vi "Set Port Interface Name.vi"(8 "error in":errorcluster, 10 "XNET Interface Name":T2, 11 "Port Ref":T1 format="%.0x") -> (0 "error out":errorcluster, 3 "Port Ref out":T1 format="%.0x")   [LabVIEW 2020, in "Communication Bus Template Scripting.lvlib"]
uses:
  <vilib>/NI VeriStand/Custom Device API/Custom Device Item Ref.ctl
  Constants.vi
  Communication Bus Template Scripting.lvlib
  <vilib>/NI VeriStand/Custom Device API/Custom Device API.lvlib
  <vilib>/NI VeriStand/Custom Device API/Set Item Property (U32).vi
  System Explorer/Implementation/System Explorer/Types/XNET Interface Name.ctl
  System Explorer/Implementation/Implementation.lvlib
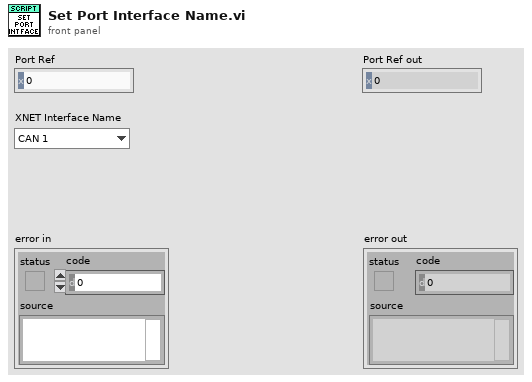
[diagram p1: front panel]
types:
  T1 = typedef "Custom Device API.lvlib/Custom Device Item Ref.ctl" = u64
  T2 = typedef "Communication Bus Template System Explorer.lvlib/Implementation.lvlib/XNET Interface Name.ctl" = enum16{"CAN 1", "CAN 2", "CAN 3", "CAN 4", "CAN 5", "CAN 6", "CAN 7", "CAN 8", "CAN 9", "CAN 10", "CAN 11", "CAN 12", "CAN 13", "CAN 14", "CAN 15", "CAN 16"}
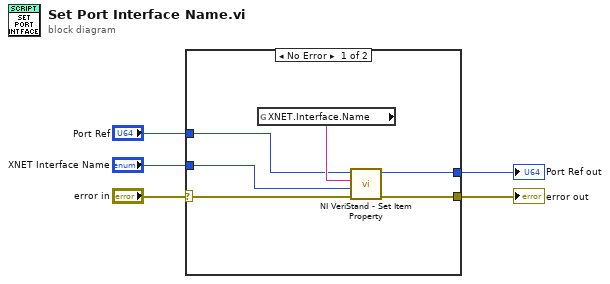
[diagram p0: block diagram]
diagram:
  n1 = case shown="No Error" "error in" {
    selector: "error in" -> [w6 w13]
    tunnel: "Port Ref" -> [w10 w12]
    tunnel: [w9 w13] -> w4
    tunnel: "XNET Interface Name" -> [w8 _]
    tunnel: [w7 w12] -> w2
    frame No Error {
      n2 = global read "Constants.vi" "XNET.Interface.Name"() -> (w11:string)
      n3 = call-poly <vilib>:"NI VeriStand - Set Item Property.vi"("error in (no error)"=w6, "Value"=w8, "Property Name"=w11, "Item Ref in"=w10) -> ("error out"=w9:errorcluster, "Item Ref out"=w7:T1)  [unwired: 5 in, 1 out]
    }
    frame Error {
    }
  }
  "error out" <- w4
  "Port Ref out" <- w2
